vi "Build ADU_TCP.vi"(8 "error in (no error)":errorcluster, 9 "Transaction ID":u16, 10 "Slave ID":u8) -> (0 "error out":errorcluster, 3 "MB_ADU_TCP out":refnum<class "MB_ADU_TCP.lvclass">)   [LabVIEW 2023, in "Jiaxin_Stepper_Controller.lvlib" / "MB Master.lvlib" / "MB_ADU_TCP.lvclass"]
uses:
  MB_ADU_TCP.lvclass
  C:/Users/quantum/Documents/LVDAQ/ConcreteClasses/ConcreteInstrumentClasses/Jiaxin_Stepper_Controller/Plasmionique/MB Master/MB_ADU/MB_ADU.lvclass
  MB_ADU/MB_ADU.lvclass/MB_ADU.ctl
  MB_ADU_TCP.lvclass/MB_ADU_TCP.ctl
  MB_ADU/MB_ADU.lvclass
panel:
  in  "MB_ADU_TCP in":refnum<class "MB_ADU_TCP.lvclass">
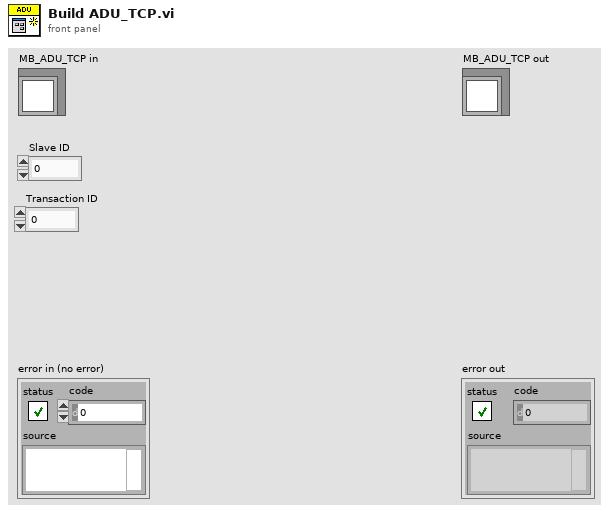
[diagram p1: front panel]
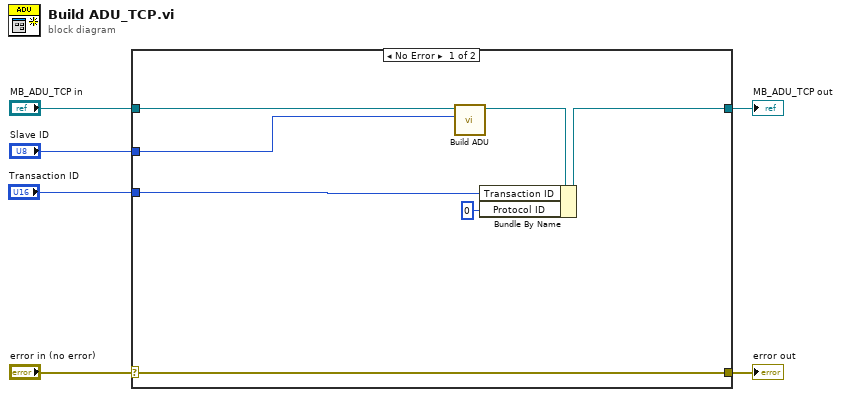
[diagram p0: block diagram]
diagram:
  n1 = case shown="No Error" "error in (no error)" {
    selector: "error in (no error)" -> [w13 w15]
    tunnel: [w13 w15] -> w5
    tunnel: [w9 w14] -> w3
    tunnel: "MB_ADU_TCP in" -> [w12 w14]
    tunnel: "Slave ID" -> [w11 _]
    tunnel: "Transaction ID" -> [w8 _]
    frame No Error {
      n2 = call "Build ADU.vi"("Slave ID"=w11, "MB_ADU in"=w12) -> ("MB_ADU out"=w10:refnum<class "MB_ADU_TCP.lvclass">)  [unwired: 8 in, 1 out]
      n3 = Bundle By Name(cluster=w10, "Transaction ID"=w8, "Protocol ID"=u16 0) -> (w9:refnum<class "MB_ADU_TCP.lvclass">)
    }
    frame Error {
    }
  }
  "error out" <- w5
  "MB_ADU_TCP out" <- w3
